vi "Forward Progress.vi"(8 "error in (no error)":errorcluster, 9 "Complete":bool, 10 "Search Label":string, 11 "BetterSearch in":refnum<class "BetterSearch.lvclass">) -> (0 "error out":errorcluster, 3 "BetterSearch out":refnum<class "BetterSearch.lvclass">)   [LabVIEW 2016, in "Better Search.lvlib" / "BetterSearch.lvclass"]
uses:
  BetterSearch.lvclass
  Search Progress.ctl
  Better Search.lvlib
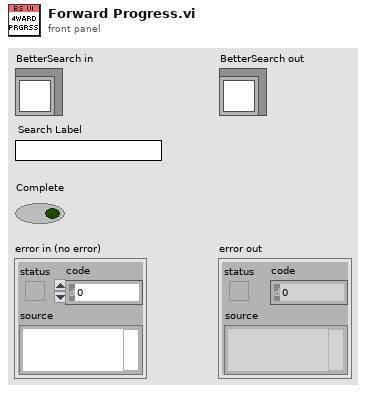
[diagram p1: front panel]
types:
  T1 = typedef "Better Search.lvlib/Search Progress.ctl" = cluster{"Complete":bool, "Label":string}
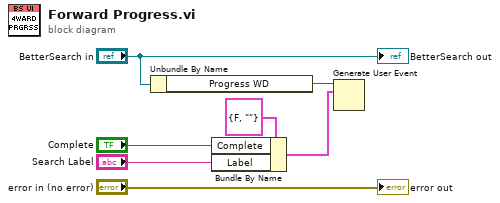
[diagram p0: block diagram]
diagram:
  n1 = Unbundle By Name("BetterSearch in") -> ("Progress WD"=w5:refnum<user-event>)
  n2 = Bundle By Name(cluster=T1 {"Complete"=FALSE, "Label"=""} ("event data"), "Complete"="Complete", "Label"="Search Label") -> (w3:T1)
  n3 = Generate User Event(user event=w5, event data cluster=w3) -> ()  [unwired: 2 in, 2 out]
  "error out" <- "error in (no error)"
  "BetterSearch out" <- "BetterSearch in"
